vi "CHS_TRAJ_BEGIN.vi"(9 "Initial Gyo Reading":T3 {"SIN" format="%13.4f"; "COS" format="%13.4f"; "VALUE" format="%13.4f"}, 10 "Robot Starting Pose":T1 {"ROTATION"."SIN" format="%13.4f"; "ROTATION"."COS" format="%13.4f"; "ROTATION"."VALUE" format="%13.4f"; "TRANSLATION"."Y" format="%14.3f"; "TRANSLATION"."X" format="%14.3f"}) -> ()   [LabVIEW 2019]
uses:
  <vilib>/Rock Robotics/WPI/ThirdParty/JAS_Junk/TrajLib/TypeDef/ROTATION2D.ctl
  <vilib>/Rock Robotics/WPI/ThirdParty/JAS_Junk/TrajLib/TypeDef/POSE2D.ctl
  <vilib>/Rock Robotics/WPI/ThirdParty/JAS_Junk/TrajLib/TypeDef/TRANSLATION2D.ctl
  CHS_TRAJECTORY_GLOBALS.vi
  <vilib>/Rock Robotics/WPI/ThirdParty/ChoreoLib/ChoreoLib.lvlib
  <vilib>/Rock Robotics/WPI/ThirdParty/JAS_Junk/TrajLib/Trajectory_Library.lvlib
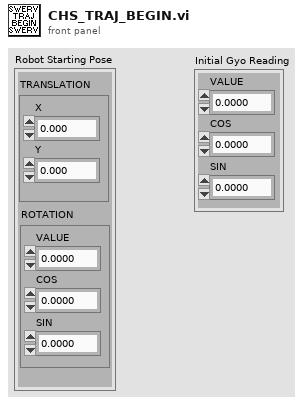
[diagram p1: front panel]
types:
  T1 = typedef "Trajectory_Library.lvlib/POSE2D.ctl" = cluster{"TRANSLATION":T2, "ROTATION":T3}
  T2 = typedef "Trajectory_Library.lvlib/TRANSLATION2D.ctl" = cluster{"X":dbl, "Y":dbl}
  T3 = typedef "Trajectory_Library.lvlib/ROTATION2D.ctl" = cluster{"VALUE":dbl, "COS":dbl, "SIN":dbl}
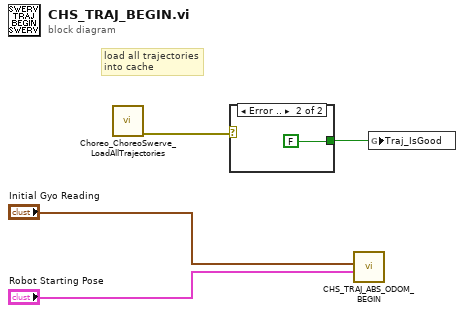
[diagram p0: block diagram]
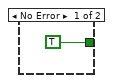
[diagram p2: hidden frame]
diagram:
  # "load all trajectories\ninto cache"
  n1 = call <vilib>:"Choreo_ChoreoSwerve_LoadAllTrajectories.vi"() -> ("error out"=w1:errorcluster)  [unwired: 11 in]
  n2 = case shown="Error .." w1 {
    tunnel: [TRUE FALSE] -> w2
    frame No Error {
    }
    frame Error {
    }
  }
  n3 = call "CHS_TRAJ_ABS_ODOM_BEGIN.vi"("Initial Pose"="Robot Starting Pose", "Initial Gyro Angle"="Initial Gyo Reading") -> ()  [unwired: 9 in, 1 out]
  n4 = global write "CHS_TRAJECTORY_GLOBALS.vi" "Traj_IsGood"(w2) -> ()
